vi "Identify.vi"(8 "error in (no error)":errorcluster, 11 "Shape in":refnum<class "Shape.lvclass">) -> (0 "error out":errorcluster, 2 "Class name":string, 3 "Shape out":refnum<class "Shape.lvclass">)   [LabVIEW 2017, in "Shape.lvclass"]
doc: "This VI is a method that demonstrates dynamic dispatching."
uses:
  Shape.lvclass
panel:
  in  "Class name (constant)":string="Shape"
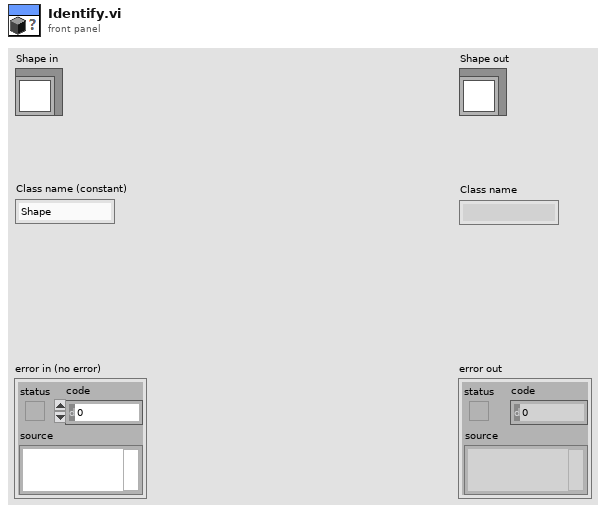
[diagram p1: front panel]
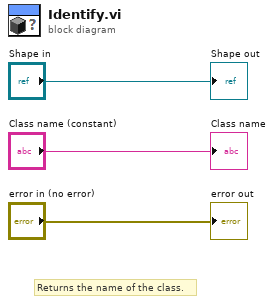
[diagram p0: block diagram]
diagram:
  # "Returns the name of the class."
  "error out" <- "error in (no error)"
  "Shape out" <- "Shape in"
  "Class name" <- "Class name (constant)"
